vi "Capture YSI.vi"(1 "Initialize":bool=TRUE, 2 "Finished In":bool, 5 "DEPTH":sgl format="%.2f", 7 "YSI Com Port":i32=2, 9 "Time Out (secs)":i32=5, 12 "Collect Ion Data":bool) -> (4 "Finished Out":bool=TRUE)   [LabVIEW 2016]
uses:
  ad interface/Global_SIM_switch.vi
  <vilib>/Utility/file.llb/Write To Spreadsheet File (DBL).vi
panel:
  out "Ion Content":dbl(graph)
  out "FLOW":dbl format="%.2f"
  out "PRESSURE":dbl format="%.2f"
  in  "Capture YSI Data":bool
  out "Specific Conductivity":dbl(graph)=16.0
  out "ORP":dbl(graph)=144.5
  out "Dissolved O2":dbl(graph)=8.51
  out "Temperature":dbl(graph)=18.76
  out "PH":dbl(graph)=8.24
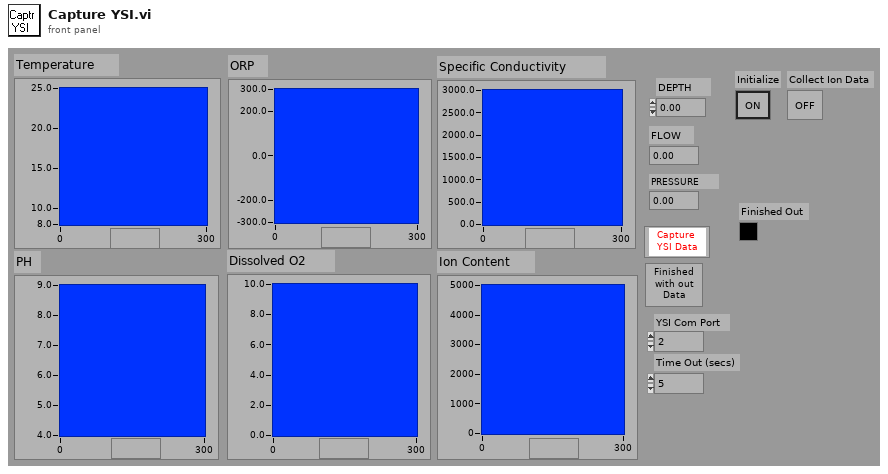
[diagram p1: front panel]
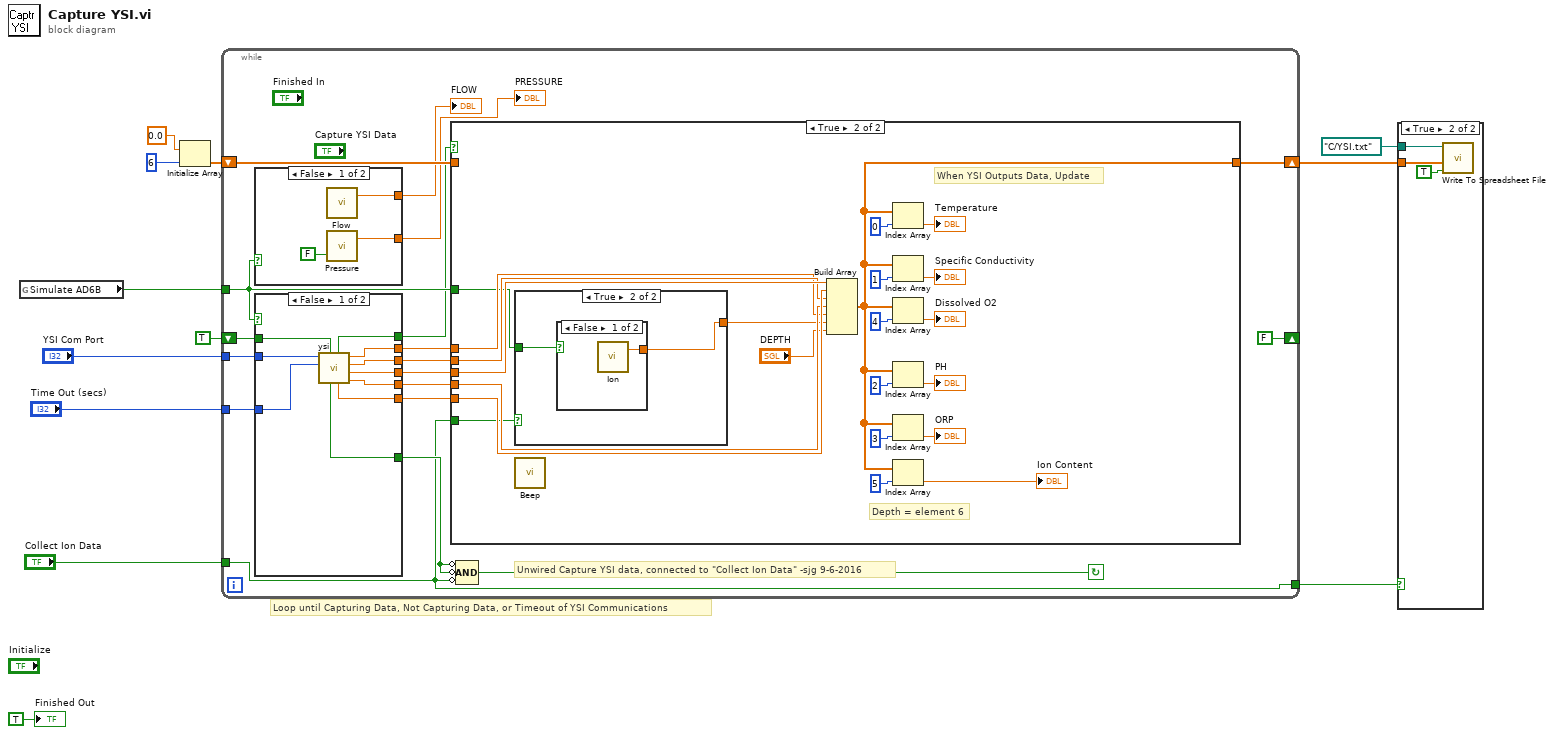
[diagram p0: block diagram]
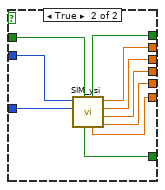
[diagram p2: hidden frame]
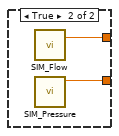
[diagram p3: hidden frame]
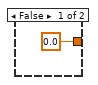
[diagram p5: hidden frame]
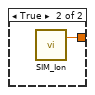
[diagram p6: hidden frame]
diagram:
  # "Loop until Capturing Data, Not Capturing Data, or Timeout of YSI Communications"
  n1 = global read "Global_SIM_switch.vi" "Simulate AD6B"() -> (w4:bool)
  n2 = Initialize Array(0.0, 6) -> (w11:dbl[])
  n3 = while {
    tunnel: w4 -> [w17]
    tunnel: "Time Out (secs)" -> [w18]
    tunnel: "YSI Com Port" -> [w19]
    tunnel: "Collect Ion Data" -> [w13]
    tunnel: [w13] -> w2
    shift-left: TRUE -> [w24]
    shift-right: [FALSE] -> _
    shift-left: w11 -> [w30]
    shift-right: [w22] -> w3
    stop <- w15 continue-if-true
    # "Unwired Capture YSI data, connected to \"Collect Ion Data\" -sjg 9-6-2016"
    n4 = case shown="False" w17 {
      tunnel: [w53 w55] -> w21
      tunnel: [w52 w54] -> w20
      frame False {
        n5 = call "Flow.vi"() -> ("Flow (ml/min)"=w53:dbl)  [unwired: 3 in]
        n6 = call "Pressure.vi"("Zero Pressure\n(F = leave as is)"=FALSE ("Zero Pressure\n(F = leave as is)")) -> ("Pressure"=w52:dbl)  [unwired: 2 in]
      }
      frame True {
        n7 = call "SIM_Flow.vi"() -> ("Flow (ml/min)"=w55:dbl)  [unwired: 3 in]
        n8 = call "SIM_Pressure.vi"() -> ("Pressure"=w54:dbl)  [unwired: 11 in]
      }
    }
    "PRESSURE" <- w20
    "FLOW" <- w21
    n9 = case shown="False" w17 {
      tunnel: [w40 w50] -> w16
      tunnel: [w39 w49] -> w29
      tunnel: [w38 w48] -> w28
      tunnel: [w37 w47] -> w27
      tunnel: [w36 w46] -> w26
      tunnel: [w35 w45] -> w25
      tunnel: w24 -> [w34 w44]
      tunnel: [w33 w43] -> w14
      tunnel: w19 -> [w32 w42]
      tunnel: w18 -> [w31 w41]
      frame False {
        n10 = call "ysi.vi"("Initialize"=w34, "Time Out (secs)"=w31, "YSI Com Port"=w32) -> ("pH"=w36:dbl, "Temperature"=w39:dbl, "dis O2"=w37:dbl, "ORP"=w35:dbl, "spec K"=w38:dbl, "Fresh Data"=w40:bool, "Time out occurred"=w33:bool)  [unwired: 2 in]
      }
      frame True {
        n11 = call "SIM_ysi.vi"("Initialize"=w44, "Time Out (secs)"=w41, "YSI Com Port"=w42) -> ("pH"=w46:dbl, "Temperature"=w49:dbl, "dis O2"=w47:dbl, "ORP"=w45:dbl, "spec K"=w48:dbl, "Fresh Data"=w50:bool, "Time out occurred"=w43:bool)  [unwired: 2 in]
      }
    }
    n12 = case shown="True" w16 {
      tunnel: w30 -> [w56 _]
      tunnel: [w56 w63] -> w22
      tunnel: w29 -> [_ w78]
      tunnel: w28 -> [_ w77]
      tunnel: w27 -> [_ w76]
      tunnel: w26 -> [_ w75]
      tunnel: w25 -> [_ w74]
      tunnel: w13 -> [_ w60]
      tunnel: w17 -> [_ w59]
      frame False {
        # "No Data Yet, No Update"
      }
      frame True {
        # "Depth = element 6"
        # "When YSI Outputs Data, Update"
        n13 = case shown="True" w60 {
          tunnel: [0.0 w81] -> w61
          tunnel: w59 -> [_ w80]
          frame False {
          }
          frame True {
            n14 = case shown="False" w80 {
              tunnel: [w82 w83] -> w81
              frame False {
                n15 = call "Ion.vi"() -> ("Ion (ppm)"=w82:dbl)  [unwired: 3 in]
              }
              frame True {
                n16 = call "SIM_Ion.vi"() -> ("Ion (ppm)"=w83:dbl)  [unwired: 3 in]
              }
            }
          }
        }
        n17 = call <vilib>:"Beep.vi"() -> ()  [unwired: 12 in]
        n18 = Build Array(w78, w77, w76, w75, w74, w61, "DEPTH") -> (w63:dbl[])
        n19 = Index Array(array=w63, index=0) -> (element=→"Temperature":dbl)
        n20 = Index Array(array=w63, index=1) -> (element=→"Specific Conductivity":dbl)
        n21 = Index Array(array=w63, index=4) -> (element=→"Dissolved O2":dbl)
        n22 = Index Array(array=w63, index=2) -> (element=→"PH":dbl)
        n23 = Index Array(array=w63, index=3) -> (element=→"ORP":dbl)
        n24 = Index Array(array=w63, index=5) -> (element=→"Ion Content":dbl)
      }
    }
    n25 = Compound Arithmetic op=AND(invert w14, invert w14, invert w13) -> (w15:bool)
  }
  n26 = case shown="True" w2 {
    tunnel: w3 -> [_ w85]
    tunnel: path "C:/YSI.txt" ("Output File") -> [_ w84]
    frame False {
    }
    frame True {
      n27 = call-poly <vilib>:"Write To Spreadsheet File.vi"("append to file? (new file:F)"=TRUE, "1D data"=w85, "file path (dialog if empty)"=w84) -> ()  [unwired: 5 in, 1 out]
    }
  }
  "Finished Out" <- TRUE
